vi "Init Task.vi"(4 "counter":tag, 6 "line grouping":i32(ring) items=["one channel for each line", "one channel for all lines"], 7 "physical channels":tag, 8 "error in (no error)":errorcluster, 9 "name":string, 10 "DAQmxTaksContainer_General":refnum<class "DAQmxTaksContainer_General.lvclass">, 11 "DAQmxTaskCounterDigital_Emulate in":refnum<class "DAQmxTaskCounterDigital_Emulate.lvclass">) -> (0 "error out":errorcluster, 3 "DAQmxTaskCounterDigital_Emulate out":refnum<class "DAQmxTaskCounterDigital_Emulate.lvclass">)   [LabVIEW 2020, in "DAQmxTaskCounterDigital_Emulate.lvclass"]
uses:
  DAQmxTaskCounterDigital_Emulate.lvclass
  C:/dev/TRANCON/Classes/DAQmxTasks/DAQmxTask.lvclass
  DAQmxTaskContainer_General/DAQmxTaksContainer_General.lvclass
  DAQmxTask.lvclass/DAQmxTask.ctl
  DAQmxTask.lvclass
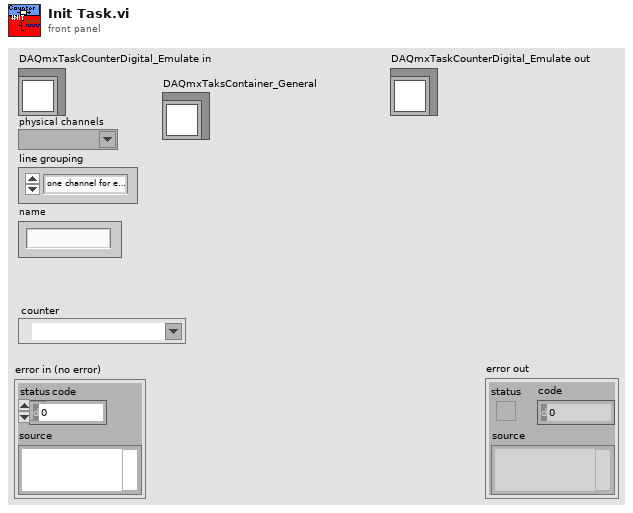
[diagram p1: front panel]
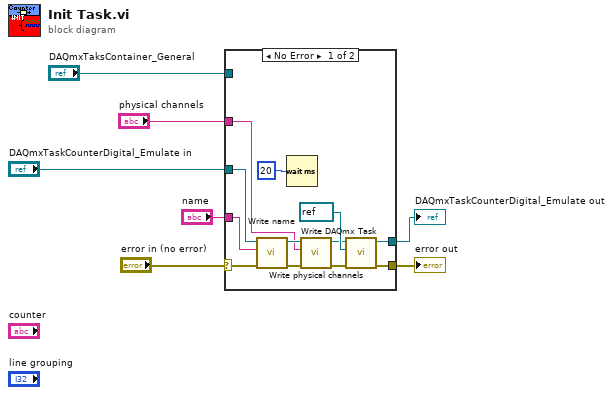
[diagram p0: block diagram]
diagram:
  n1 = case shown="No Error" "error in (no error)" {
    selector: "error in (no error)" -> [w14 w21]
    tunnel: "name" -> [w10 _]
    tunnel: "DAQmxTaskCounterDigital_Emulate in" -> [w13 w20]
    tunnel: [w9 w21] -> w7
    tunnel: "physical channels" -> [w12 _]
    tunnel: "DAQmxTaksContainer_General" -> [_ _]
    tunnel: [w8 w20] -> w1
    frame No Error {
      n2 = call "Write name.vi"("error in (no error)"=w14, "name"=w10, "DAQmxTask in"=w13) -> ("error out"=w16:errorcluster, "DAQmxTask out"=w17:refnum<class "DAQmxTaskCounterDigital_Emulate.lvclass">)  [unwired: 7 in]
      n3 = Wait (ms)(milliseconds to wait=u32 20) -> ()  [unwired: 1 out]
      n4 = call "Write physical channels.vi"("error in (no error)"=w16, "physical channels"=w12, "DAQmxTask in"=w17) -> ("error out"=w15:errorcluster, "DAQmxTask out"=w18:refnum<class "DAQmxTaskCounterDigital_Emulate.lvclass">)  [unwired: 7 in]
      n5 = call "Write DAQmx Task.vi"("error in (no error)"=w15, "DAQmx Task Name"=refnum<k21> refnum, "DAQmxTask in"=w18) -> ("error out"=w9:errorcluster, "DAQmxTask out"=w8:refnum<class "DAQmxTaskCounterDigital_Emulate.lvclass">)  [unwired: 7 in]
    }
    frame Error {
    }
  }
  "error out" <- w7
  "DAQmxTaskCounterDigital_Emulate out" <- w1
